vi "program.vi"() -> ()   [LabVIEW 2020]
uses:
  <vilib>/Instr/_visa.llb/VISA Configure Serial Port (Instr).vi
panel:
  out "Log Data":string[][](table)
  out "Name":string
  out "UID":string
  in  "VISA resource name":refnum<visa-resource-name>
  in  "stop":bool
  # "SCAN"
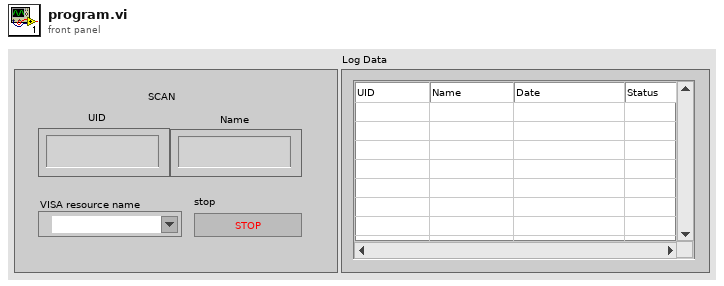
[diagram p1: front panel]
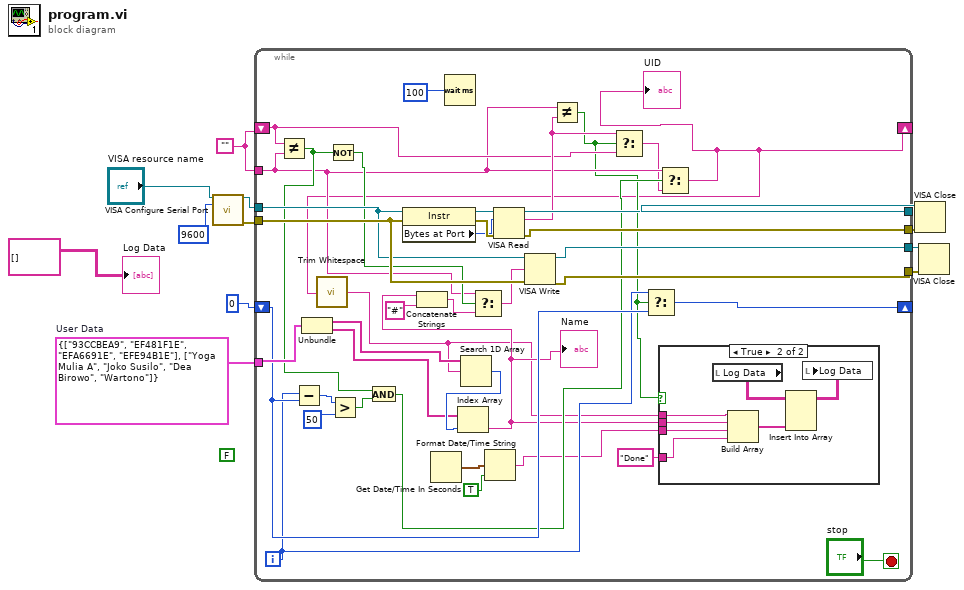
[diagram p0: block diagram]
diagram:
  (unwired) FALSE
  w3 = cluster{string[], string[]} {["93CCBEA9", "EF481F1E", "EFA6691E", "EFE94B1E"], ["Yoga Mulia A", "Joko Susilo", "Dea Birowo", "Wartono"]}  # User Data
  w4 = ""
  n1 = call-poly "VISA Configure Serial Port"("VISA resource name"="VISA resource name", "baud rate (9600)"=u32 9600) -> ("VISA resource name out"=w7:refnum<visa-resource-name>, "error out"=w10:errorcluster)  [unwired: 12 in]
  n2 = while {
    tunnel: w7 -> [w42]
    tunnel: w10 -> [w43]
    tunnel: [w47] -> w9
    tunnel: [w46] -> w8
    shift-right: [w17] -> _
    shift-left: w4 -> [w35]
    tunnel: [w41] -> w6
    tunnel: [w40] -> w5
    tunnel: w4 -> [w26]
    tunnel: w3 -> [w36]
    shift-right: [w30] -> _
    shift-left: 0 -> [w29]
    i -> [w28]
    stop <- "stop" stop-if-true
    n3 = Not Equal?(x=w35, y=w26) -> (x != y?=w33:bool)
    n4 = Subtract(x=w28, y=w29) -> (x-y=w24:i32)
    n5 = Unbundle(w36) -> (w23:string[], w21:string[])
    n6 = Not(x=w33) -> (.not. x?=w34:bool)
    n7 = Greater?(x=w24, y=50) -> (0:w31:bool)
    n8 = And(x=w33, y=w31) -> (x .and. y?=w27:bool)
    n9 = property class="Instr"(reference=w42, error in=w43) -> (reference out=w49:refnum<visa-resource-name>, error out=w50:errorcluster, "Bytes at Port"=w48:u32)
    n10 = Get Date/Time In Seconds() -> (seconds since 1Jan1904=w15:timestamp)
    n11 = Wait (ms)(milliseconds to wait=u32 100) -> ()  [unwired: 1 out]
    n12 = Format Date/Time String(seconds (now)=w15, UTC format=TRUE) -> (date/time string=w14:string)  [unwired: 1 in]
    n13 = VISA Read(VISA resource name=w49, byte count=w48, error in (no error)=w50) -> (VISA resource name out=w47:refnum<visa-resource-name>, read buffer=w44:string, error out=w46:errorcluster)  [unwired: 1 out]
    n14 = Not Equal?(x=w26, y=w44) -> (x != y?=w19:bool)
    n15 = Select(t=w44, s=w19, f=w35) -> (s? t:f=w25:string)
    n16 = Select(t=w28, s=w19, f=w29) -> (s? t:f=w30:i32)
    n17 = Select(t=w26, s=w27, f=w25) -> (s? t:f=w17:string)
    "UID" <- w17
    n18 = call <vilib>:"Trim Whitespace.vi"("string"=w17) -> ("trimmed string"=w16:string)  [unwired: 1 in]
    n19 = Search 1D Array(1D array=w23, element=w16) -> (index of element=w22:i32)  [unwired: 1 in]
    n20 = Index Array(array=w21, index=w22) -> (element=w20:string)
    "Name" <- w20
    n21 = Concatenate Strings(w20, "#" ("string")) -> (w38:string)
    n22 = Select(t=w26, s=w34, f=w38) -> (s? t:f=w37:string)
    n23 = VISA Write(VISA resource name=w42, write buffer=w37, error in (no error)=w43) -> (VISA resource name out=w41:refnum<visa-resource-name>, error out=w40:errorcluster)  [unwired: 1 out]
    n24 = case shown="True" w19 {
      tunnel: w16 -> [_ w56]
      tunnel: w20 -> [_ w55]
      tunnel: "Done" ("new element/subarray") -> [_ w53]
      tunnel: w14 -> [_ w52]
      frame False {
      }
      frame True {
        n25 = local read "Log Data"() -> (w57:string[][])
        n26 = Build Array(w56, w55, w52, w53) -> (w54:string[])
        n27 = Insert Into Array(array=w57, new element=w54) -> (w58:string[][])  [unwired: 2 in]
        n28 = local write "Log Data"(w58) -> ()
      }
    }
  }
  n29 = VISA Close(VISA resource name=w9, error in (no error)=w8) -> ()  [unwired: 1 out]
  n30 = VISA Close(VISA resource name=w6, error in (no error)=w5) -> ()  [unwired: 1 out]
  "Log Data" <- string[][] []
